vi "Read Timing Data (Go Down and Dispense).vi"(8 "error in (no error)":errorcluster, 11 "Dispense in":refnum<class "Dispense.lvclass">) -> (0 "error out":errorcluster, 2 "Timing Data (Go Down and Dispense)":T1(array[cluster]), 3 "Dispense out":refnum<class "Dispense.lvclass">)   [LabVIEW 2016, in "Dispense.lvclass"]
uses:
  Dispense.lvclass
  Dispense.lvclass/Dispense.ctl
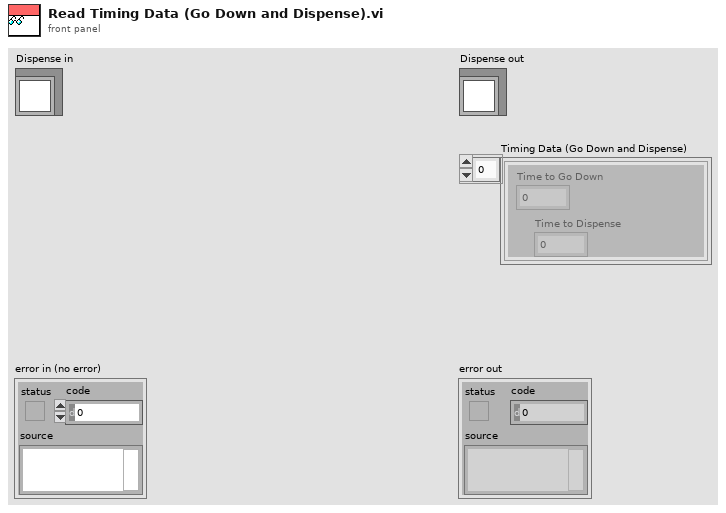
[diagram p1: front panel]
types:
  T1 = cluster{"Time to Go Down":dbl, "Time to Dispense":dbl}[]
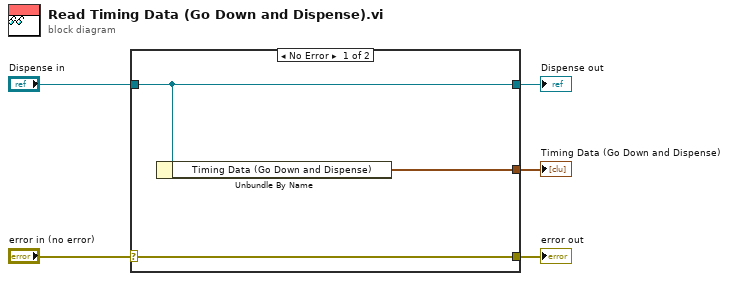
[diagram p0: block diagram]
diagram:
  n1 = case shown="No Error" "error in (no error)" {
    selector: "error in (no error)" -> [w8 w9]
    tunnel: [w8 w9] -> w4
    tunnel: [w7 w10] -> w2
    tunnel: "Dispense in" -> [w7 w10]
    tunnel: [w6 _] -> w1
    frame No Error {
      n2 = Unbundle By Name(w7) -> ("Timing Data (Go Down and Dispense)"=w6:T1)
    }
    frame Error {
    }
  }
  "error out" <- w4
  "Dispense out" <- w2
  "Timing Data (Go Down and Dispense)" <- w1
